vi "fgv_obstacle_data.vi"(7 "cmd":T1=enum."read", 8 "error in":errorcluster, 9 "inrange pt-n":u32, 10 "obstacle in":bool=TRUE, 11 "limit in":cluster{"RL range":dbl, "Point limit":u16} {"Point limit" scale=0.0..10.0; "RL range" scale=0.0..10.0}) -> (0 "error out":errorcluster, 1 "inrange pt-n out":u32, 2 "obstacle out":bool, 3 "limit out":cluster{"RL range":dbl, "Point limit":u16} {"Point limit" scale=0.0..10.0; "RL range" scale=0.0..10.0})   [LabVIEW 2019]
uses:
  Ctrl/obstacle_info.ctl
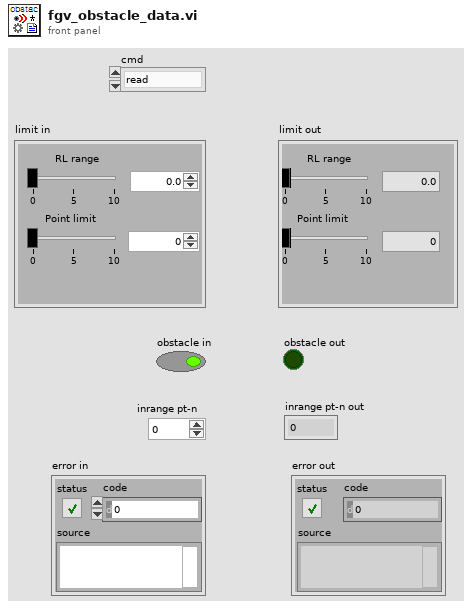
[diagram p1: front panel]
types:
  T1 = typedef "obstacle_info.ctl" = enum16{"init", "read", "obstacle status in", "write limit", "inrange pt-n"}
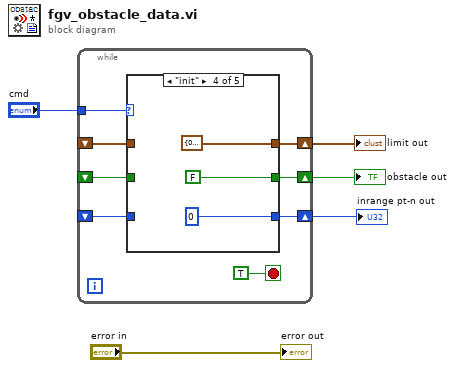
[diagram p0: block diagram]
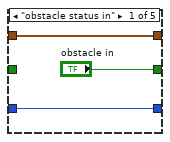
[diagram p2: hidden frame]
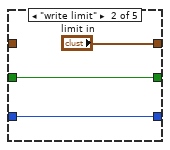
[diagram p3: hidden frame]
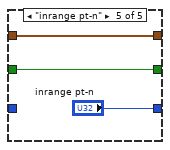
[diagram p5: hidden frame]
diagram:
  n1 = while {
    shift-right: [w11] -> w2
    shift-left: _ -> [w10]
    tunnel: "cmd" -> [w12]
    shift-right: [w9] -> w4
    shift-left: _ -> [w8]
    shift-right: [w7] -> w1
    shift-left: _ -> [w6]
    stop <- TRUE stop-if-true
    n2 = case shown="\"init\"" w12 {
      tunnel: [w16 "limit in" w22 cluster{"RL front-x":dbl, "RL central-x":u16} {"RL front-x"=0.0, "RL central-x"=0} ("limit range") w27] -> w11
      tunnel: w10 -> [w16 _ w22 _ w27]
      tunnel: ["obstacle in" w19 w21 FALSE ("obstacle in") w28] -> w9
      tunnel: w8 -> [_ w19 w21 _ w28]
      tunnel: [w14 w17 w20 u32 0 ("inrange pt-n") "inrange pt-n"] -> w7
      tunnel: w6 -> [w14 w17 w20 _ _]
      frame "obstacle status in" {
      }
      frame "write limit" {
      }
      frame "read", Default {
      }
      frame "init" {
      }
      frame "inrange pt-n" {
      }
    }
  }
  "obstacle out" <- w4
  "limit out" <- w2
  "inrange pt-n out" <- w1
  "error out" <- "error in"
